vi "averagebackground.vi"(0 "Input Array":dbl[][](array[numeric])=[[0.0, 0.0, 0.0, 0.0, 0.0, 0.0, 0.0, 0.0, 0.0, 0.0, 0.0, 1.0], [0.0, 1.0, 0.0, 0.0, 0.0, 0.0, 0.0, 0.0, 0.0, 0.0, 2.0, 0.0], [0.0, 0.0, 2.0, 0.0, 0.0, 0.0, 0.0, 0.0, 0.0, 3.0, 0.0, 0.0], [0.0, 0.0, 0.0, 3.0, 0.0, 0.0, 0.0, 0.0, 4.0, 0.0, 0.0, 0.0], [0.0, 0.0, 0.0, 0.0, 4.0, 0.0, 0.0, 5.0, 0.0, 0.0, 0.0, 0.0], [0.0, 0.0, 0.0, 0.0, 0.0, 5.0, 6.0, 0.0, 0.0, 0.0, 0.0, 0.0], [0.0, 0.0, 0.0, 0.0, 0.0, 7.0, 6.0, 0.0, 0.0, 0.0, 0.0, 0.0], [3.0, 0.0, 0.0, 0.0, 8.0, 0.0, 0.0, 7.0, 0.0, 0.0, 0.0, 0.0], [0.0, 2.0, 0.0, 9.0, 0.0, 0.0, 0.0, 0.0, 8.0, 0.0, 8.0, 7.0], [3.0, 0.0, 1.0, 0.0, 0.0, 0.0, 0.0, 0.0, 0.0, 9.0, 0.0, 2.0]] format="%.2f") -> (1 "sum of Gaussian":dbl format="%.2f", 2 "average # of counts in corner areas":dbl format="%.2f")   [LabVIEW 2013]
doc: "This VI calculates the average number of counts per pixel for a background area (the corners). Then, it calculates what the total number of counts in the entire array would be if there were no atoms. It subtracts this number from the total # of actual counts in the entire array. Notes on p. 71 of Pascal's Lab Notebook #3."
panel:
  out "total number of pixels multiplied\nby average count/pixel":dbl format="%.2f"
  in  "percentage of dimension to use as corner":dbl=0.1 format="%.2f"
  out "sum of counts in all pixels":dbl format="%.2f"
  out "bottom right":dbl[][](array[numeric]) format="%.2f"
  out "top right":dbl[][](array[numeric]) format="%.2f"
  out "bottom left":dbl[][](array[numeric]) format="%.2f"
  out "top left":dbl[][](array[numeric]) format="%.2f"
  out "# of x pixels to use in corner":dbl format="%.2f"
  out "# of y pixels to use in corner":dbl format="%.2f"
  out "x size":i32
  out "y size":i32
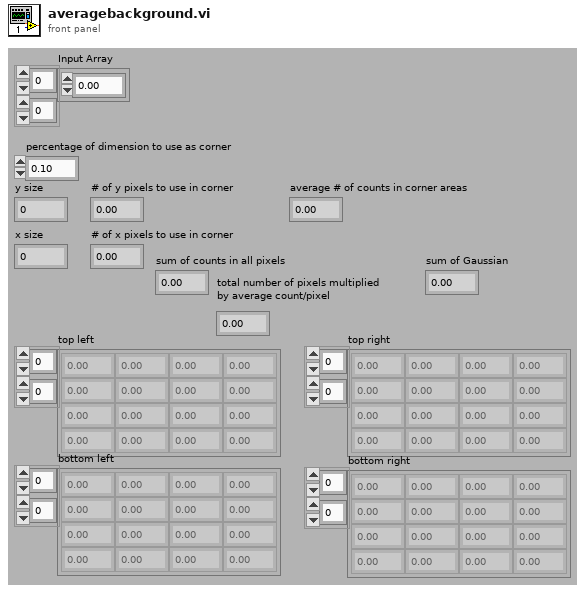
[diagram p1: front panel]
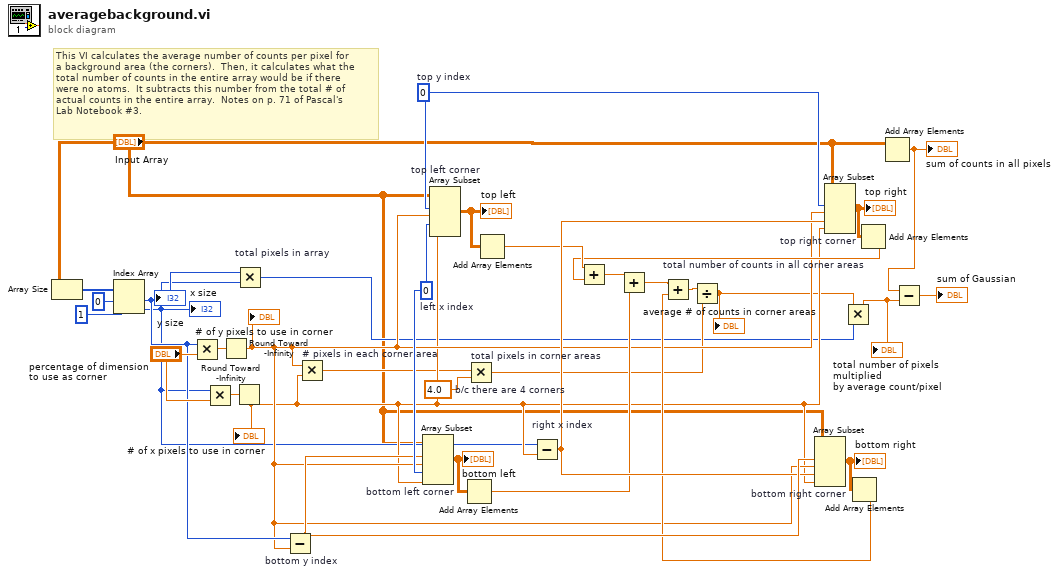
[diagram p0: block diagram]
diagram:
  w9 = 4.0  # b/c there are 4 corners
  w28 = 0  # left x index
  w26 = 0  # top y index
  # "This VI calculates the average number of counts per pixel for\na background area (the corners).  Then, it calculates what the\ntotal number of counts in the entire array would be if there\nwere no atoms.  It subtracts this number from the total # of\nactual counts in the entire array.  Notes on p. 71 of Pascal's\nLab Notebook #3."
  n1 = Array Size(array="Input Array") -> (size(s)=w34:i32[])
  n2 = Index Array "Index Array"(array=w34, index #1=0 ("index"), index #2=1 ("index")) -> (element #1=w23:i32, element #2=w6:i32)
  "y size" <- w23
  "x size" <- w6
  n3 = Multiply(x=w23, y="percentage of dimension to use as corner") -> (x*y=w31:dbl)
  n4 = Multiply(x=w6, y="percentage of dimension to use as corner") -> (x*y=w29:dbl)
  n5 = Round Toward -Infinity(1:w31) -> (0:w12:dbl)
  "# of y pixels to use in corner" <- w12
  n6 = Round Toward -Infinity(1:w29) -> (0:w11:dbl)
  "# of x pixels to use in corner" <- w11
  n7 = Multiply "total pixels in array"(x=w23, y=w6) -> (x*y=w3:i32)
  n8 = Subtract "bottom y index"(x=w23, y=w12) -> (x-y=w25:dbl)
  n9 = Multiply "# pixels in each corner area"(x=w12, y=w11) -> (x*y=w10:dbl)
  n10 = Array Subset "bottom left corner"(array="Input Array", index (row)=w25, length (row)=w12, index (col)=w28, length (col)=w11) -> (w21:dbl[][])
  "bottom left" <- w21
  n11 = Array Subset "top left corner"(array="Input Array", index (row)=w26, length (row)=w12, index (col)=w28, length (col)=w11) -> (w27:dbl[][])
  "top left" <- w27
  n12 = Add Array Elements(numeric array=w21) -> (sum=w16:dbl)
  n13 = Multiply "total pixels in corner areas"(x=w10, y=w9) -> (x*y=w8:dbl)
  n14 = Add Array Elements(numeric array=w27) -> (sum=w19:dbl)
  n15 = Subtract "right x index"(x=w6, y=w11) -> (x-y=w24:dbl)
  n16 = Array Subset "bottom right corner"(array="Input Array", index (row)=w25, length (row)=w12, index (col)=w24, length (col)=w11) -> (w22:dbl[][])
  "bottom right" <- w22
  n17 = Array Subset "top right corner"(array="Input Array", index (row)=w26, length (row)=w12, index (col)=w24, length (col)=w11) -> (w20:dbl[][])
  "top right" <- w20
  n18 = Add Array Elements(numeric array=w22) -> (sum=w14:dbl)
  n19 = Add Array Elements(numeric array=w20) -> (sum=w18:dbl)
  n20 = Add(x=w19, y=w18) -> (x+y=w17:dbl)
  n21 = Add(x=w17, y=w16) -> (x+y=w15:dbl)
  n22 = Add "total number of counts in all corner areas"(x=w15, y=w14) -> (x+y=w13:dbl)
  n23 = Divide(x=w13, y=w8) -> (x/y=w4:dbl)
  "average # of counts in corner areas" <- w4
  n24 = Multiply(x=w4, y=w3) -> (x*y=w2:dbl)
  "total number of pixels multiplied\nby average count/pixel" <- w2
  n25 = Add Array Elements(numeric array="Input Array") -> (sum=w7:dbl)
  "sum of counts in all pixels" <- w7
  n26 = Subtract(x=w7, y=w2) -> (x-y=→"sum of Gaussian":dbl)
